vi "Add User To Database.vi"(4 "Name(\"\")":string, 6 "Pwd(\"\")":string, 7 "Table(\"\")":string, 8 "error in (no error)":errorcluster, 9 "ID(\"\")":string, 10 "UserName(\"\")":string, 11 "Login in":refnum<class "Login.lvclass">) -> (0 "error out":errorcluster, 3 "Login out":refnum<class "Login.lvclass">)   [LabVIEW 2015, in "Login.lvclass"]
uses:
  Login.lvclass
  Login.lvclass/Login.ctl
  API/_Database/Database.lvclass
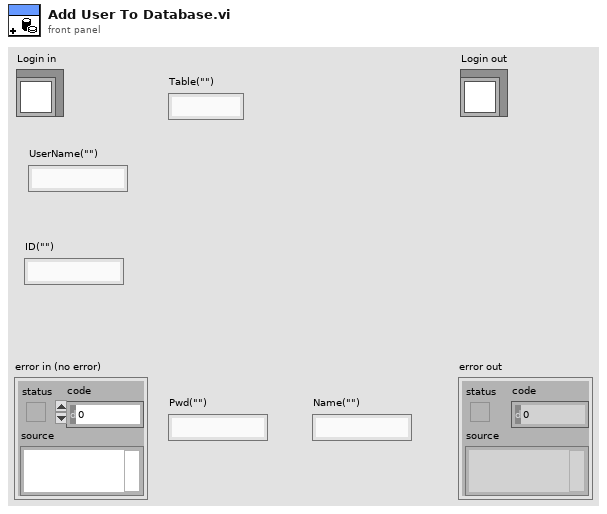
[diagram p1: front panel]
types:
  T1 = cluster{"UserName(\"\")":string, "Name(\"\") ":string, "ID(\"\")":string, "Pwd(\"\")":string}
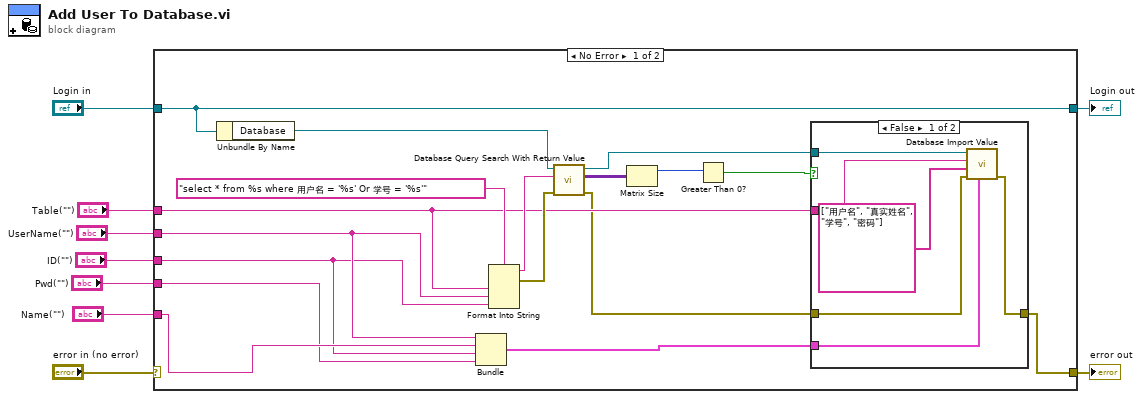
[diagram p0: block diagram]
diagram:
  n1 = case shown="No Error" "error in (no error)" {
    selector: "error in (no error)" -> [_ w35]
    tunnel: [w14 w35] -> w8
    tunnel: [w26 w34] -> w6
    tunnel: "Login in" -> [w26 w34]
    tunnel: "UserName(\"\")" -> [w16 _]
    tunnel: "ID(\"\")" -> [w11 _]
    tunnel: "Pwd(\"\")" -> [w10 _]
    tunnel: "Table(\"\")" -> [w17 _]
    tunnel: "Name(\"\")" -> [w12 _]
    frame No Error {
      n2 = Unbundle By Name(w26) -> ("Database"=w19:refnum<class "Database.lvclass">)
      n3 = Bundle("UserName(\"\")"=w16, "Name(\"\")"=w12, "ID(\"\")"=w11, "Pwd(\"\")"=w10) -> (w15:T1)  [unwired: 1 in]
      n4 = Format Into String(format string="select * from %s where 用户名 = '%s' Or 学号 = '%s'", w17, w16, w11) -> (resulting string=w24:string, error out=w23:errorcluster)  [unwired: 2 in]
      n5 = call "Database Query Search With Return Value.vi"("error in (no error)"=w23, "SQL query"=w24, "object in"=w19) -> ("error out"=w13:errorcluster, "recordset data"=w21:variant[][], "object out"=w18:refnum<class "Database.lvclass">)  [unwired: 5 in, 1 out]
      n6 = Matrix Size(0:w21) -> (1:w22:i32)  [unwired: 1 out]
      n7 = Greater Than 0?(x=w22) -> (x > 0?=w20:bool)
      n8 = case shown="False" w20 {
        tunnel: w18 -> [w32 _]
        tunnel: w13 -> [w28 w33]
        tunnel: w17 -> [w31 _]
        tunnel: w15 -> [w29 _]
        tunnel: [w27 w33] -> w14
        frame False {
          n9 = call "Database Import Value.vi"("data"=w29, "error in (no error)"=w28, "columns"=string[] ["用户名", "真实姓名", "学号", "密码"], "table"=w31, "object in"=w32) -> ("error out"=w27:errorcluster)  [unwired: 5 in, 1 out]
        }
        frame True {
        }
      }
    }
    frame Error {
    }
  }
  "error out" <- w8
  "Login out" <- w6
